vi "Insert Bus Monitor.vi"(8 "error in (no error)":errorcluster, 10 "Protected Subpanel":T1, 11 "Mediator in":refnum<class "Mediator.lvclass">) -> (0 "error out":errorcluster, 3 "Mediator out":refnum<class "Mediator.lvclass">)   [LabVIEW 2017, in "MyMediator.lvlib副本.lvlib" / "Mediator.lvclass"]
uses:
  Mediator.lvclass
  <vilib>/Composed/GPM Packages/mva-framework/Source/Framework/IViewable/ProtectedSubpanel/Protected Subpanel Reference.ctl
  <vilib>/Composed/GPM Packages/mva-framework/Source/Framework/IViewable/ProtectedSubpanel/ProtectedSubpanel.lvclass
  Mediator.lvclass/Mediator.ctl
  <vilib>/Composed/GPM Packages/mva-framework/Source/Framework/IViewable/IViewable Messages/Insert Front Panel Msg/Insert Front Panel Msg.lvclass/Insert Front Panel Msg.ctl
  <vilib>/ActorFramework/Message Enqueuer/Message Enqueuer.lvclass/Message Enqueuer.ctl
  <vilib>/ActorFramework/Message Enqueuer/Enqueue.vi
  <vilib>/Composed/GPM Packages/mva-framework/Source/Framework/IViewable/IViewable Messages/Insert Front Panel Msg/Insert Front Panel Msg.lvclass
  C:/Program Files (x86)/National Instruments/LabVIEW 2017/vi.lib/ActorFramework/Message/Message.lvclass
  <vilib>/ActorFramework/Message Priority Queue/Priority Enqueue.vi
  <vilib>/ActorFramework/Message Enqueuer/Message Enqueuer.lvclass
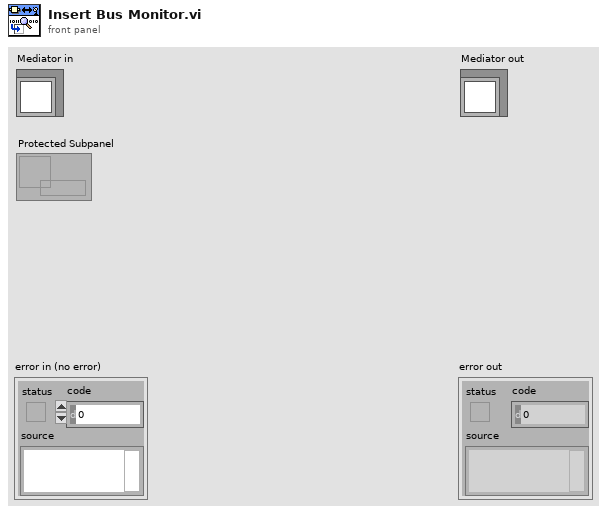
[diagram p1: front panel]
types:
  T1 = typedef "IViewable.lvlib/ProtectedSubpanel.lvclass/Protected Subpanel Reference.ctl" = refnum<data-value>
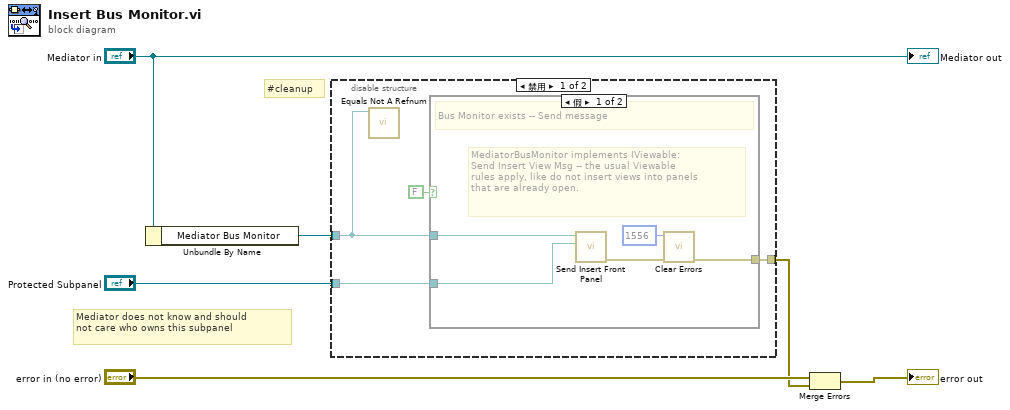
[diagram p0: block diagram]
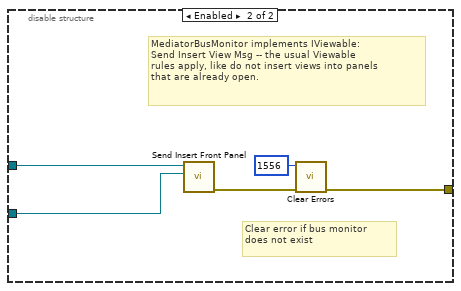
[diagram p3: hidden frame]
diagram:
  # "#cleanup"
  # "Mediator does not know and should\nnot care who owns this subpanel"
  n1 = Unbundle By Name("Mediator in") -> ("Mediator Bus Monitor"=w1:refnum<class "Message Enqueuer.lvclass">)
  n2 = disable-structure shown="禁用" {
    disable-tunnel: "Protected Subpanel" -> [w10 w17]
    disable-tunnel: [w9 w16] -> w2
    disable-tunnel: w1 -> [w8 w18]
    frame Disabled {
      n3 = call <vilib>:"Equals Not A Refnum.vi"("Message Enqueuer"=w8) -> ()  [unwired: 10 in, 1 out]
      n4 = case shown="假" FALSE {
        tunnel: w8 -> [w15 _]
        tunnel: w10 -> [w14 _]
        tunnel: [w13 _] -> w9
        frame False {
          # "MediatorBusMonitor implements IViewable:\nSend Insert View Msg -- the usual Viewable\nrules apply, like do not insert views into panels\nthat are already open."
          # "Bus Monitor exists -- Send message"
          n5 = call <vilib>:"Send Insert Front Panel.vi"("Protected Subpanel"=w14, "Message Enqueuer"=w15) -> ("error out"=w12:errorcluster)  [unwired: 8 in, 1 out]
          n6 = call <vilib>:"Clear Errors.vi"("error in (no error)"=w12, "specific error code to clear (0: all)"=1556) -> ("error out"=w13:errorcluster)  [unwired: 4 in, 1 out]
        }
        frame True {
          # "No Bus Monitor -- Send nothing"
        }
      }
    }
    frame Enabled {
      # "Clear error if bus monitor\ndoes not exist"
      # "MediatorBusMonitor implements IViewable:\nSend Insert View Msg -- the usual Viewable\nrules apply, like do not insert views into panels\nthat are already open."
      n7 = call <vilib>:"Send Insert Front Panel.vi"("Protected Subpanel"=w17, "Message Enqueuer"=w18) -> ("error out"=w20:errorcluster)  [unwired: 8 in, 1 out]
      n8 = call <vilib>:"Clear Errors.vi"("error in (no error)"=w20, "specific error code to clear (0: all)"=1556) -> ("error out"=w16:errorcluster)  [unwired: 4 in, 1 out]
    }
  }
  n9 = Merge Errors("error in (no error)", w2) -> (→"error out":errorcluster)
  "Mediator out" <- "Mediator in"
